vi "CtrlHandler.Mathematica.vi"(0 "Data":variant, 1 "Type":T1=enum."Value Change", 2 "Ctrl":refnum<vi>, 3 "Name":string) -> ()   [LabVIEW 2014]
uses:
  <vilib>/event_ctls.llb/lveventtype.ctl
  E:/Mathematica/Wolfram.NETLink.dll
  Mathematica/Wolfram.NETLink.dll
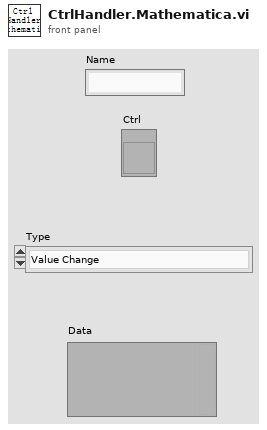
[diagram p1: front panel]
types:
  T1 = typedef "lveventtype.ctl" = enum32{"Null", "Timeout", "Annotation Menu Selection", "Annotation Menu Selection?", "App Instance Close", "App Instance Close?", "Autoscale Range Change", "Bookmark Info Change", "Cell Edit", "Cell Edit?", "Cursor Grab", "Cursor Grab?", "Cursor Menu Selection", "Cursor Menu Selection?", "Cursor Move", "Cursor Release", "Data Change", "Direction Change", "Display State Change", "Drag Ended", "Drag Enter", "Drag Leave", "Drag Over", "Drag Source Update", "Drag Starting", "Drag Starting?", "Drop", "Exec State Change", "Key Down", "Key Down?", "Key Repeat", "Key Repeat?", "Key Up", "Listbox Double Click", "Menu Activation?", "Menu Selection (App)", "Menu Selection? (App)", "Menu Selection (User)", "Mouse Down", "Mouse Down?", "Mouse Enter", "Mouse Leave", "Mouse Move", "Mouse Up", "Mouse Wheel", "NI Security User Change (App)", "Pane Size", "Panel Close", "Panel Close?", "Panel Resize", "Plot Attribute Change", "Scale Range Change", "Shortcut Menu Activation?", "Shortcut Menu Selection (App)", "Shortcut Menu Selection? (App)", "Shortcut Menu Selection (User)", "Tree Double Click", "Tree Drag", "Tree Drag?", "Tree Drop", "Tree Drop?", "Tree Item Close", "Tree Item Close?", "Tree Item Open", "Tree Item Open?", "User Event", "Value Change"}
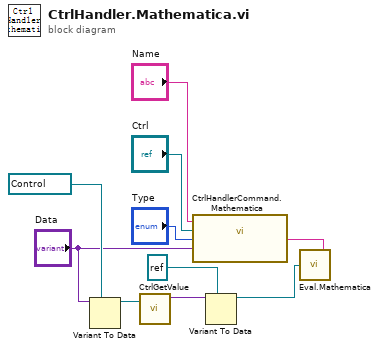
[diagram p0: block diagram]
diagram:
  n1 = Variant To Data(type=refnum<vi> refnum ("Ctrl"), Variant="Data") -> (data=w1:refnum<vi>)  [unwired: 1 in, 1 out]
  n2 = call "CtrlGetValue.vi"("reference"=w1) -> ("variant"=w4:variant)  [unwired: 1 in, 3 out]
  n3 = call "CtrlHandlerCommand.Mathematica.vi"("Data"="Data", "Type"="Type", "Ctrl"="Ctrl", "Name"="Name") -> ("Command"=w5:string)
  n4 = Variant To Data(type=refnum<k24> refnum ("Mathematica"), Variant=w4) -> (data=w6:refnum<k24>)  [unwired: 1 in, 1 out]
  n5 = call "Eval.Mathematica.vi"("input"=w5, "reference"=w6) -> ()
